vi "waitXms.vi"(2 "attente (ms)":u32, 7 "errin":errorcluster) -> (8 "errout":errorcluster)   [LabVIEW 2020]
doc: "Ce Vi fait perdre 50ms"
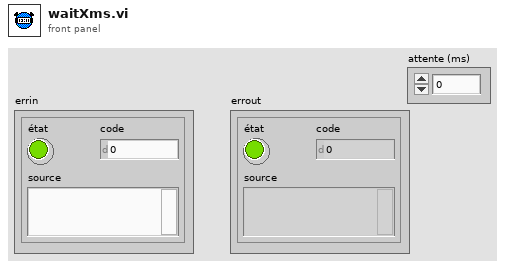
[diagram p1: front panel]
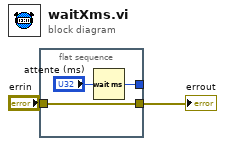
[diagram p0: block diagram]
diagram:
  n1 = flat-sequence {
    tunnel: [w5] -> _
    tunnel: "errin" -> [w4]
    tunnel: [w4] -> w2
    frame #0 {
      n2 = Wait (ms)(milliseconds to wait="attente (ms)") -> (millisecond timer value=w5:u32)
    }
  }
  "errout" <- w2
